vi "PC-FP-Elements-FGV - Kopie.vi"(0 "VI-ref":refnum<vi>, 5 "Name":string, 7 "Value in":string, 9 "Mode":T2(ring), 11 "error in":errorcluster) -> (4 "ElementRef.":refnum<vi>, 6 "Datatype":string, 8 "Value out":string, 10 "Cluster":T1, 15 "error out":errorcluster)   [LabVIEW 2016]
uses:
  <vilib>/ErrorRing/Error Ring.xnode
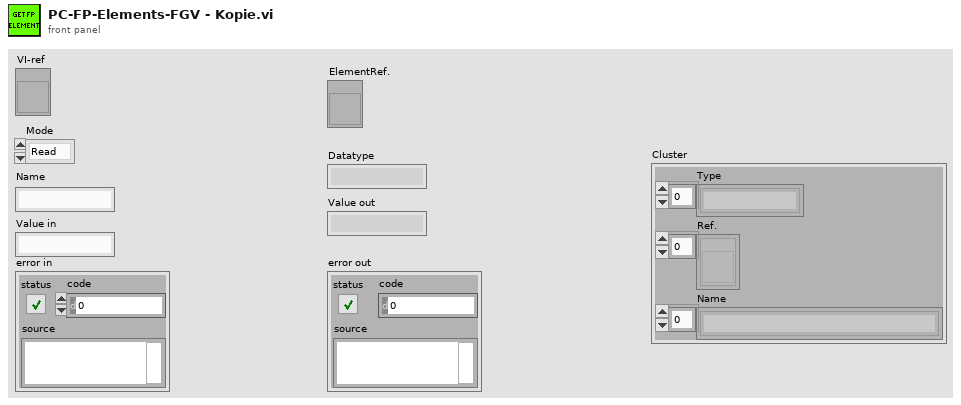
[diagram p1: front panel]
types:
  T1 = cluster{"Type":string[], "Ref.":refnum<vi>[], "Name":string[]}
  T2 = enum16{"Read", "Delete", "SetElement", "GetElement", "GetFPelements"}
  T3 = typedef "LVNumericRepresentation.ctl" = enum32{"Extended Precision", "Double Precision", "Single Precision", "Long", "Word", "Byte", "Unsigned Long", "Unsigned Word", "Unsigned Byte", "Complex Extended", "Complex Double", "Complex Single", "Quad", "Unsigned Quad", "Fixed-Point"}
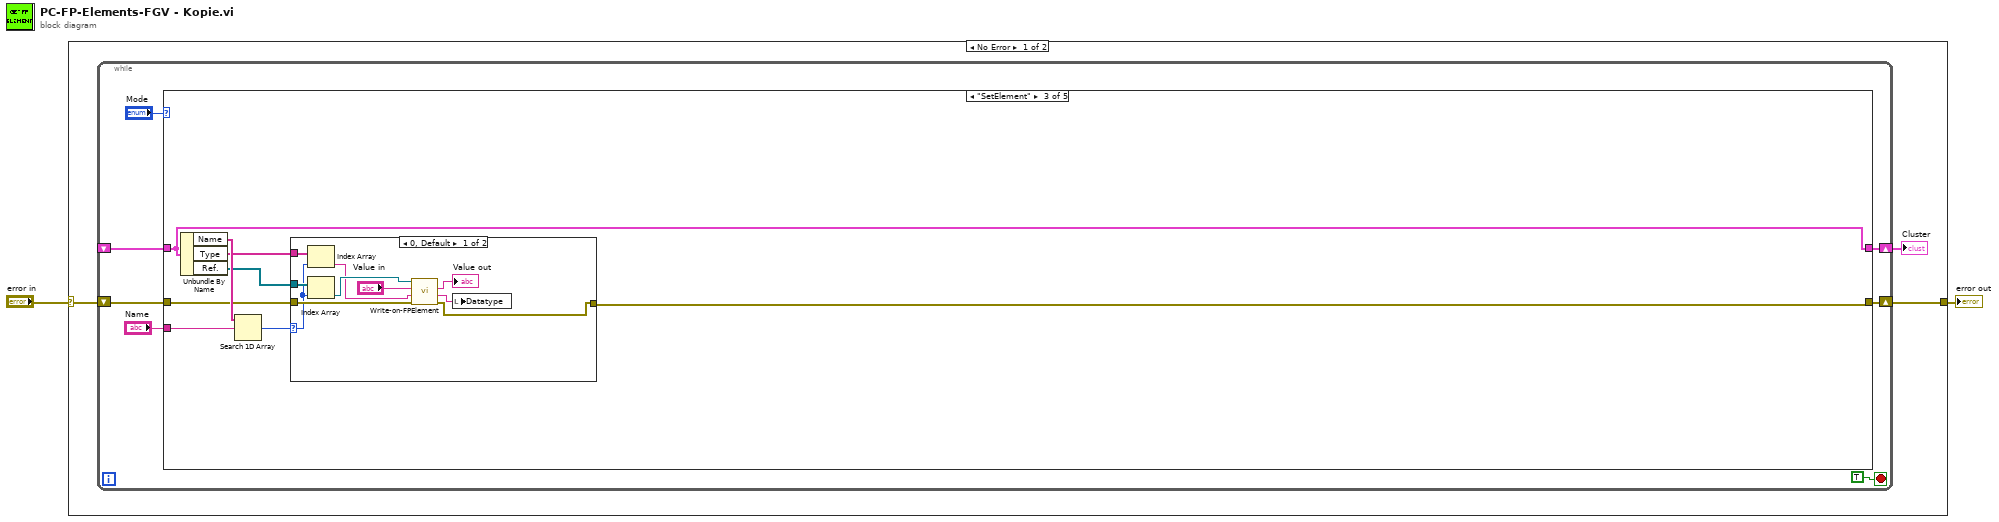
[diagram p0: block diagram]
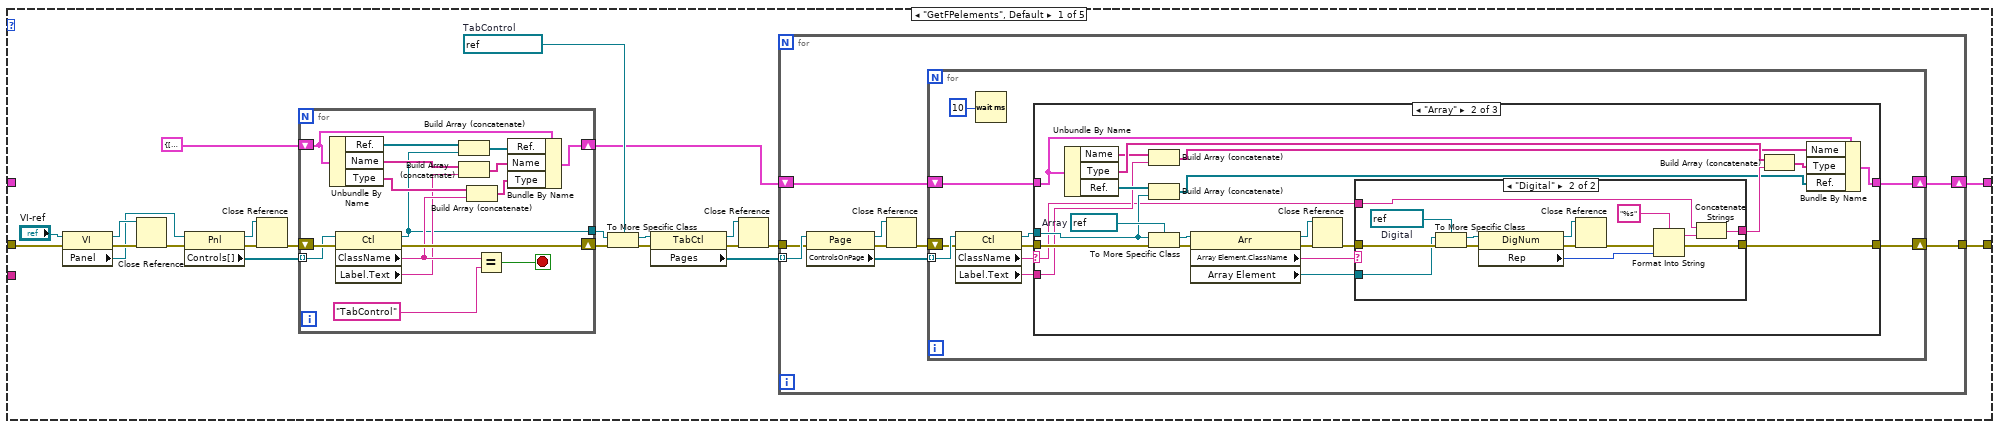
[diagram p2: hidden frame]
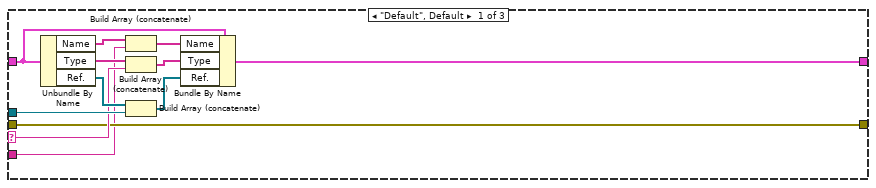
[diagram p3: hidden frame]
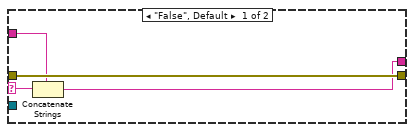
[diagram p4: hidden frame]
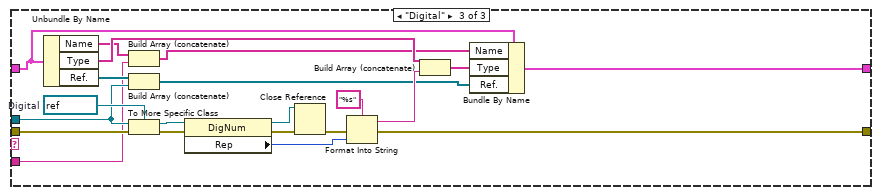
[diagram p5: hidden frame]
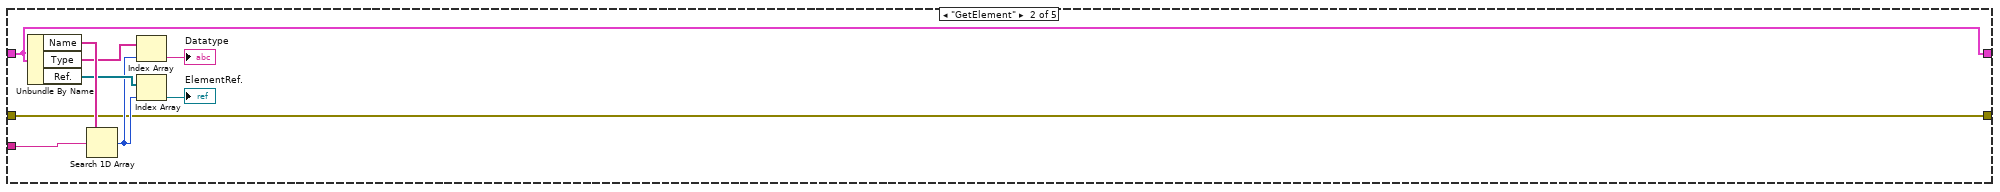
[diagram p6: hidden frame]
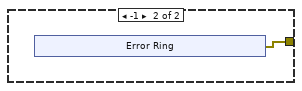
[diagram p7: hidden frame]
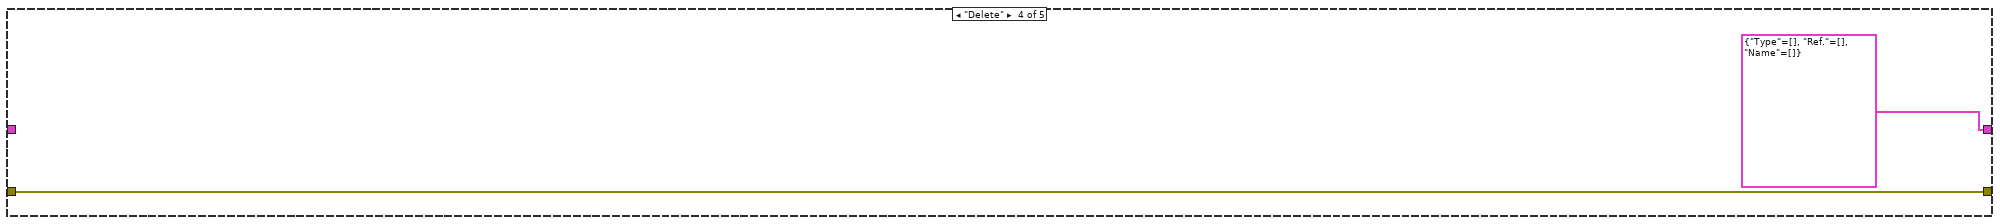
[diagram p8: hidden frame]
diagram:
  n1 = case shown="No Error" "error in" {
    selector: "error in" -> [w3 w177]
    tunnel: [w5 w177] -> w2
    frame No Error {
      n2 = while {
        shift-right: [w11] -> w4
        shift-left: _ -> [w10]
        shift-right: [w7] -> w5
        shift-left: w3 -> [w8]
        stop <- TRUE stop-if-true
        n3 = case shown="\"SetElement\"" "Mode" {
          tunnel: [w28 w147 w157 T1 {"Type"=[], "Ref."=[], "Name"=[]} w175] -> w11
          tunnel: w10 -> [_ w147 w157 _ w175]
          tunnel: w8 -> [w27 w145 w155 w173 w176]
          tunnel: [w26 w145 w153 w173 w176] -> w7
          tunnel: "Name" -> [_ w144 w156 _ _]
          frame "GetFPelements", Default {
            w21 = refnum<vi> refnum  # TabControl
            n4 = property class="VI"(reference="VI-ref", error in=w27) -> (reference out=w32:refnum<vi>, error out=w34:errorcluster, "Panel"=w31:refnum<vi>)
            n5 = Close Reference(reference=w32, error in (no error)=w34) -> (error out=w33:errorcluster)
            n6 = property class="Pnl"(reference=w31, error in=w33) -> (reference out=w29:refnum<vi>, error out=w30:errorcluster, "Controls[]"=w24:refnum<vi>[])
            n7 = Close Reference(reference=w29, error in (no error)=w30) -> (error out=w25:errorcluster)
            n8 = for {
              tunnel: w24 -> [w46] mode=indexing
              shift-right: [w48] -> w22
              shift-left: w25 -> [w51]
              tunnel: [w36] -> w23
              shift-right: [w37] -> w13
              shift-left: T1 {"Type"=[], "Ref."=[], "Name"=[]} -> [w41]
              stop <- w49 stop-if-true
              n9 = Unbundle By Name(w41) -> ("Ref."=w47:refnum<vi>[], "Name"=w45:string[], "Type"=w44:string[])
              n10 = property class="Ctl"(reference=w46, error in=w51) -> (reference out=w36:refnum<vi>, error out=w48:errorcluster, "ClassName"=w43:string, "Label.Text"=w42:string)
              n11 = Build Array (concatenate)(w47, w36) -> (w40:refnum<vi>[])
              n12 = Build Array (concatenate)(w45, w42) -> (w39:string[])
              n13 = Build Array (concatenate)(w44, w43) -> (w38:string[])
              n14 = Equal?(x=w43, y="TabControl" ("Class Name")) -> (x = y?=w49:bool)
              n15 = Bundle By Name(cluster=w41, "Ref."=w40, "Name"=w39, "Type"=w38) -> (w37:T1)
            }
            n16 = To More Specific Class(target class=w21, reference=w23, error in=w22) -> (specific class reference=w20:refnum<vi>, error out=w19:errorcluster)
            n17 = property class="TabCtl"(reference=w20, error in=w19) -> (reference out=w15:refnum<vi>, error out=w17:errorcluster, "Pages"=w18:refnum<vi>[])
            n18 = Close Reference(reference=w15, error in (no error)=w17) -> (error out=w16:errorcluster)
            n19 = for {
              tunnel: [w59] -> w26
              shift-right: [w60] -> w28
              shift-left: w13 -> [w58]
              tunnel: w18 -> [w57] mode=indexing
              tunnel: w16 -> [w56]
              n20 = property class="Page"(reference=w57, error in=w56) -> (reference out=w52:refnum<vi>, error out=w55:errorcluster, "ControlsOnPage"=w54:refnum<vi>[])
              n21 = Close Reference(reference=w52, error in (no error)=w55) -> (error out=w53:errorcluster)
              n22 = for {
                tunnel: w54 -> [w70] mode=indexing
                shift-right: [w64] -> w60
                shift-left: w58 -> [w65]
                shift-right: [w62] -> w59
                shift-left: w53 -> [w69]
                n23 = property class="Ctl"(reference=w70, error in=w69) -> (reference out=w67:refnum<vi>, error out=w66:errorcluster, "ClassName"=w68:string, "Label.Text"=w63:string)
                n24 = Wait (ms)(milliseconds to wait=u32 10) -> ()  [unwired: 1 out]
                n25 = case shown="\"Array\"" w68 {
                  selector: w68 -> [w75 w83 _]
                  tunnel: w67 -> [w77 w92 w129]
                  tunnel: w66 -> [w74 w104 w135]
                  tunnel: w65 -> [w81 w100 w131]
                  tunnel: [w82 w101 w127] -> w64
                  tunnel: w63 -> [w71 w88 w123]
                  tunnel: [w74 w87 w126] -> w62
                  frame "Default", Default {
                    n26 = Unbundle By Name(w81) -> ("Name"=w72:string[], "Type"=w80:string[], "Ref."=w78:refnum<vi>[])
                    n27 = Build Array (concatenate)(w72, w71) -> (w73:string[])
                    n28 = Build Array (concatenate)(w80, w75) -> (w79:string[])
                    n29 = Build Array (concatenate)(w78, w77) -> (w76:refnum<vi>[])
                    n30 = Bundle By Name(cluster=w81, "Name"=w73, "Type"=w79, "Ref."=w76) -> (w82:T1)
                  }
                  frame "Array" {
                    w102 = refnum<vi> refnum  # Array
                    n31 = Unbundle By Name(w100) -> ("Name"=w89:string[], "Type"=w97:string[], "Ref."=w94:refnum<vi>[])
                    n32 = Build Array (concatenate)(w89, w88) -> (w90:string[])
                    n33 = Build Array (concatenate)(w94, w92) -> (w91:refnum<vi>[])
                    n34 = To More Specific Class(target class=w102, reference=w92, error in=w104) -> (specific class reference=w93:refnum<vi>, error out=w103:errorcluster)
                    n35 = property class="Arr"(reference=w93, error in=w103) -> (reference out=w84:refnum<vi>, error out=w98:errorcluster, "Array Element.ClassName"=w99:string, "Array Element"=w86:refnum<vi>)
                    n36 = Close Reference(reference=w84, error in (no error)=w98) -> (error out=w85:errorcluster)
                    n37 = case shown="\"Digital\"" w99 {
                      selector: w99 -> [w108 _]
                      tunnel: w85 -> [w107 w120]
                      tunnel: [w106 w114] -> w96
                      tunnel: [w107 w111] -> w87
                      tunnel: w86 -> [_ w110]
                      tunnel: w83 -> [w105 w109]
                      frame "False", Default {
                        n38 = Concatenate Strings(w105, w108) -> (w106:string)
                      }
                      frame "Digital" {
                        w122 = refnum<vi> refnum  # Digital
                        n39 = To More Specific Class(target class=w122, reference=w110, error in=w120) -> (specific class reference=w121:refnum<vi>, error out=w119:errorcluster)
                        n40 = property class="DigNum"(reference=w121, error in=w119) -> (reference out=w112:refnum<vi>, error out=w116:errorcluster, "Rep"=w117:T3)
                        n41 = Close Reference(reference=w112, error in (no error)=w116) -> (error out=w113:errorcluster)
                        n42 = Format Into String(format string="%s", error in=w113, w117) -> (resulting string=w115:string, error out=w111:errorcluster)  [unwired: 1 in]
                        n43 = Concatenate Strings(w109, w115) -> (w114:string)
                      }
                    }
                    n44 = Build Array (concatenate)(w97, w96) -> (w95:string[])
                    n45 = Bundle By Name(cluster=w100, "Name"=w90, "Type"=w95, "Ref."=w91) -> (w101:T1)
                  }
                  frame "Digital" {
                    w143 = refnum<vi> refnum  # Digital
                    n46 = Unbundle By Name(w131) -> ("Name"=w125:string[], "Type"=w134:string[], "Ref."=w132:refnum<vi>[])
                    n47 = Build Array (concatenate)(w125, w123) -> (w124:string[])
                    n48 = Build Array (concatenate)(w132, w129) -> (w128:refnum<vi>[])
                    n49 = To More Specific Class(target class=w143, reference=w129, error in=w135) -> (specific class reference=w142:refnum<vi>, error out=w141:errorcluster)
                    n50 = property class="DigNum"(reference=w142, error in=w141) -> (reference out=w136:refnum<vi>, error out=w138:errorcluster, "Rep"=w139:T3)
                    n51 = Close Reference(reference=w136, error in (no error)=w138) -> (error out=w137:errorcluster)
                    n52 = Format Into String(format string="%s", error in=w137, w139) -> (resulting string=w130:string, error out=w126:errorcluster)  [unwired: 1 in]
                    n53 = Build Array (concatenate)(w134, w130) -> (w133:string[])
                    n54 = Bundle By Name(cluster=w131, "Name"=w124, "Type"=w133, "Ref."=w128) -> (w127:T1)
                  }
                }
              }
            }
          }
          frame "GetElement" {
            n55 = Unbundle By Name(w147) -> ("Name"=w152:string[], "Type"=w151:string[], "Ref."=w150:refnum<vi>[])
            n56 = Search 1D Array(1D array=w152, element=w144) -> (index of element=w149:i32)  [unwired: 1 in]
            n57 = Index Array(array=w151, index=w149) -> (element=→"Datatype":string)
            n58 = Index Array(array=w150, index=w149) -> (element=→"ElementRef.":refnum<vi>)
          }
          frame "SetElement" {
            n59 = Unbundle By Name(w157) -> ("Name"=w160:string[], "Type"=w159:string[], "Ref."=w158:refnum<vi>[])
            n60 = Search 1D Array(1D array=w160, element=w156) -> (index of element=w154:i32)  [unwired: 1 in]
            n61 = case shown="0, Default" w154 {
              selector: w154 -> [w162 _]
              tunnel: w159 -> [w170 _]
              tunnel: w158 -> [w169 _]
              tunnel: w155 -> [w167 _]
              tunnel: [w161 w171] -> w153
              frame 0, Default {
                n62 = Index Array(array=w170, index=w162) -> (element=w166:string)
                n63 = Index Array(array=w169, index=w162) -> (element=w168:refnum<vi>)
                n64 = call "Write-on-FPElement.vi"("error in (no error)"=w167, "Data type in"=w166, "Value in"="Value in", "Control in"=w168) -> ("error out"=w161:errorcluster, "Data type out"=w164:string, "Value out"=→"Value out":string)  [unwired: 4 in, 1 out]
                n65 = local write "Datatype"(w164) -> ()
              }
              frame -1 {
                n66 = xnode "Error Ring"() -> ("error out"=w171:errorcluster)
              }
            }
          }
          frame "Delete" {
          }
          frame "Read" {
          }
        }
      }
      "Cluster" <- w4
    }
    frame Error {
    }
  }
  "error out" <- w2
